vi "J-KEM July 2016.vi"(7 "Control temp?":bool, 8 "Set temp (C)":dbl format="%#_3f", 10 "Address in":T1, 11 "J-KEM on?":bool) -> (0 "current temp string":string, 1 "Current temp (C)":dbl format="%#_6f", 2 "Address out":T1, 3 "Current setpoint (C)":dbl)   [LabVIEW 2014]
uses:
  <vilib>/Instr/_visa.llb/VISA Flush IO Buffer Mask.ctl
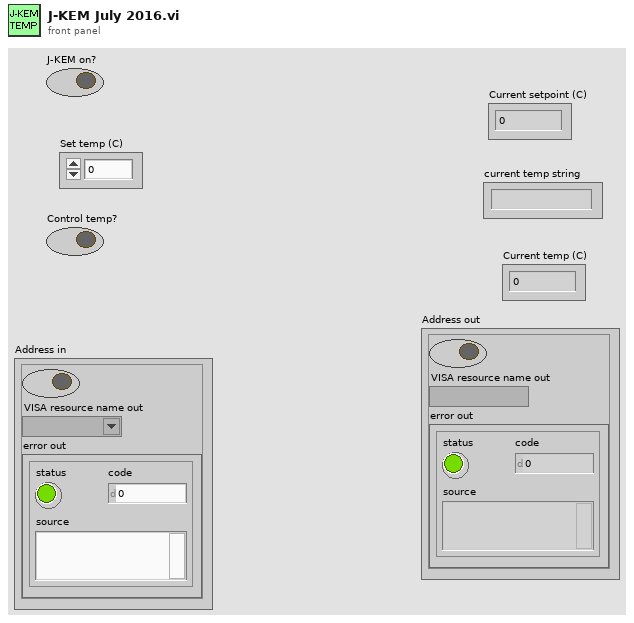
[diagram p1: front panel]
types:
  T1 = cluster{"Boolean":bool, "VISA resource name out":refnum<visa-resource-name>, "error out":errorcluster}
  T2 = typedef "VISA Flush IO Buffer Mask.ctl" = u16
  T3 = cluster{bool, "VISA Refnum out":refnum<visa-resource-name>, "error out":errorcluster}
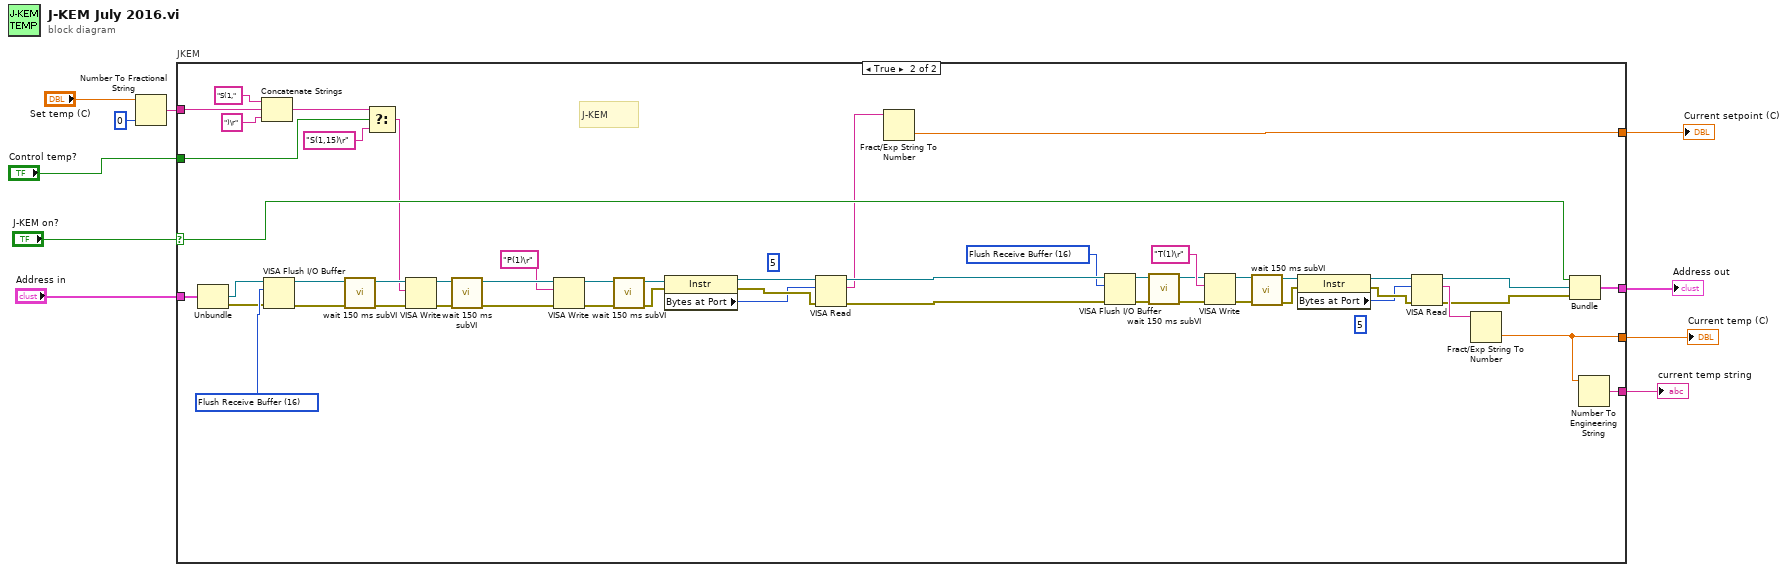
[diagram p0: block diagram]
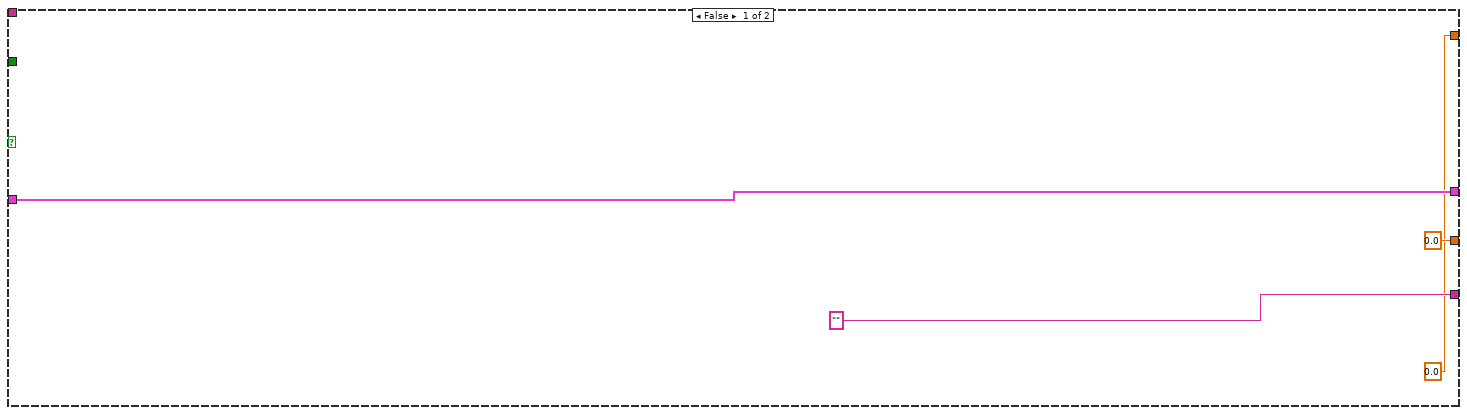
[diagram p2: hidden frame]
diagram:
  n1 = Number To Fractional String(number="Set temp (C)", precision (6)=i16 0) -> (F-format string=w4:string)  [unwired: 2 in]
  n2 = case "JKEM" shown="True" "J-KEM on?" {
    selector: "J-KEM on?" -> [_ w62]
    tunnel: "Address in" -> [w14 w65]
    tunnel: [w14 w64] -> w7
    tunnel: ["" w63] -> w8
    tunnel: w4 -> [_ w59]
    tunnel: "Control temp?" -> [_ w16]
    tunnel: [0.0 w35] -> w2
    tunnel: [0.0 w15] -> w1
    frame False {
    }
    frame True {
      (unwired) u32 5 ("byte count")
      w37 = T2 16 items=["Flush Receive Buffer"=16, "Write Transmit Buffer to Device"=32, "Flush Receive Buffer (No I/O)"=64, "Flush Transmit Buffer"=128] ("Mask")
      (unwired) u32 5 ("byte count")
      w58 = T2 16 items=["Flush Receive Buffer"=16, "Write Transmit Buffer to Device"=32, "Flush Receive Buffer (No I/O)"=64, "Flush Transmit Buffer"=128] ("Mask")
      # "J-KEM"
      n3 = Unbundle(w65) -> ("VISA resource name out"=w57:refnum<visa-resource-name>, "error out"=w56:errorcluster)  [unwired: 1 out]
      n4 = Concatenate Strings("S(1," ("write buffer"), w59, ")\r" ("write buffer")) -> (w19:string)
      n5 = VISA Flush I/O Buffer(VISA resource name=w57, mask (16)=w58, error in (no error)=w56) -> (VISA resource name out=w47:refnum<visa-resource-name>, error out=w46:errorcluster)
      n6 = call "wait 150 ms subVI.vi"("error in (no error)"=w46, "VISA Refnum in"=w47) -> ("error out"=w25:errorcluster, "VISA Refnum out"=w26:refnum<visa-resource-name>)  [unwired: 8 in]
      n7 = Select(t=w19, s=w16, f="S(1,15)\r" ("write buffer")) -> (s? t:f=w18:string)
      n8 = VISA Write(VISA resource name=w26, write buffer=w18, error in (no error)=w25) -> (VISA resource name out=w33:refnum<visa-resource-name>, error out=w30:errorcluster)  [unwired: 1 out]
      n9 = call "wait 150 ms subVI.vi"("error in (no error)"=w30, "VISA Refnum in"=w33) -> ("error out"=w31:errorcluster, "VISA Refnum out"=w32:refnum<visa-resource-name>)  [unwired: 8 in]
      n10 = VISA Write(VISA resource name=w32, write buffer="P(1)\r", error in (no error)=w31) -> (VISA resource name out=w24:refnum<visa-resource-name>, error out=w21:errorcluster)  [unwired: 1 out]
      n11 = call "wait 150 ms subVI.vi"("error in (no error)"=w21, "VISA Refnum in"=w24) -> ("error out"=w20:errorcluster, "VISA Refnum out"=w23:refnum<visa-resource-name>)  [unwired: 8 in]
      n12 = property class="Instr"(reference=w23, error in=w20) -> (reference out=w28:refnum<visa-resource-name>, error out=w27:errorcluster, "Bytes at Port"=w22:u32)
      n13 = VISA Read(VISA resource name=w28, byte count=w22, error in (no error)=w27) -> (VISA resource name out=w38:refnum<visa-resource-name>, read buffer=w34:string, error out=w39:errorcluster)  [unwired: 1 out]
      n14 = Fract/Exp String To Number(string=w34) -> (number=w15:dbl)  [unwired: 3 in, 1 out]
      n15 = VISA Flush I/O Buffer(VISA resource name=w38, mask (16)=w37, error in (no error)=w39) -> (VISA resource name out=w41:refnum<visa-resource-name>, error out=w40:errorcluster)
      n16 = call "wait 150 ms subVI.vi"("error in (no error)"=w40, "VISA Refnum in"=w41) -> ("error out"=w50:errorcluster, "VISA Refnum out"=w51:refnum<visa-resource-name>)  [unwired: 8 in]
      n17 = VISA Write(VISA resource name=w51, write buffer="T(1)\r", error in (no error)=w50) -> (VISA resource name out=w45:refnum<visa-resource-name>, error out=w43:errorcluster)  [unwired: 1 out]
      n18 = call "wait 150 ms subVI.vi"("error in (no error)"=w43, "VISA Refnum in"=w45) -> ("error out"=w42:errorcluster, "VISA Refnum out"=w44:refnum<visa-resource-name>)  [unwired: 8 in]
      n19 = property class="Instr"(reference=w44, error in=w42) -> (reference out=w52:refnum<visa-resource-name>, error out=w53:errorcluster, "Bytes at Port"=w36:u32)
      n20 = VISA Read(VISA resource name=w52, byte count=w36, error in (no error)=w53) -> (VISA resource name out=w49:refnum<visa-resource-name>, read buffer=w54:string, error out=w48:errorcluster)  [unwired: 1 out]
      n21 = Fract/Exp String To Number(string=w54) -> (number=w35:dbl)  [unwired: 3 in, 1 out]
      n22 = Bundle(w62, "VISA Refnum out"=w49, "error out"=w48) -> (w64:T3)  [unwired: 1 in]
      n23 = Number To Engineering String(4:w35) -> (0:w63:string)  [unwired: 3 in]
    }
  }
  "current temp string" <- w8
  "Address out" <- w7
  "Current temp (C)" <- w2
  "Current setpoint (C)" <- w1
